vi "Initialize Master.vi"(8 "error in (no error)":errorcluster, 11 "TCP master in":refnum<class "TCP Master.lvclass">) -> (0 "error out":errorcluster, 3 "TCP master out":refnum<class "TCP Master.lvclass">)   [LabVIEW 2018, in "SubVIs.lvlib" / "TCP Master.lvclass"]
doc: "Opens a TCP connection to the address and port stored in the class."
uses:
  TCP Master.lvclass
  TCP Master.lvclass/TCP Master.ctl
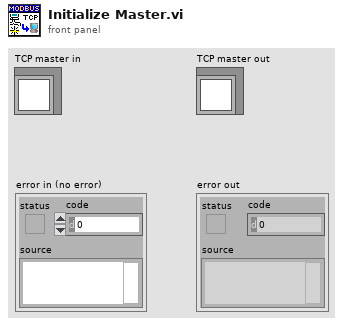
[diagram p1: front panel]
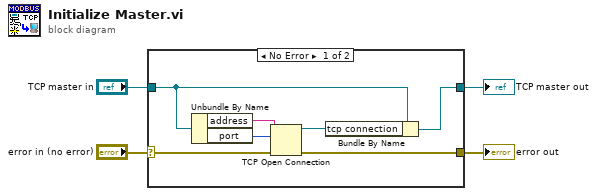
[diagram p0: block diagram]
diagram:
  n1 = case shown="No Error" "error in (no error)" {
    selector: "error in (no error)" -> [w5 w12]
    tunnel: [w9 w12] -> w4
    tunnel: "TCP master in" -> [w8 w13]
    tunnel: [w6 w13] -> w2
    frame No Error {
      n2 = Unbundle By Name(w8) -> ("address"=w11:string, "port"=w10:u16)
      n3 = TCP Open Connection(address=w11, remote port or service name=w10, error in (no error)=w5) -> (connection ID=w7:refnum<k5>, error out=w9:errorcluster)  [unwired: 2 in]
      n4 = Bundle By Name(cluster=w8, "tcp connection"=w7) -> (w6:refnum<class "TCP Master.lvclass">)
    }
    frame Error {
    }
  }
  "error out" <- w4
  "TCP master out" <- w2
